vi "kuirs_LMS_滤除指定频率干扰_1.vi"() -> ()   [LabVIEW 2017]
uses:
  <vilib>/addons/Adaptive Filters/Create/AFT Create FIR LMS (Real).vi
  <vilib>/addons/Adaptive Filters/Processing/AFT Filter Signal and Update Coefficients (Real, Array).vi
  <vilib>/addons/Adaptive Filters/Analysis/AFT Get Coefficients (FIR, Real).vi
  <vilib>/Analysis/NI_AALBase.lvlib
  <vilib>/addons/Adaptive Filters/NI_AdaptiveFilter.lvlib
panel:
  out "max step":dbl
  out "coefficient":dbl[](graph)
  in  "干扰幅值":dbl(slide)=17.0 scale=0.1..2.0
  in  "噪声标准差":dbl(slide)=17.0 scale=0.0..3.0
  in  "信号周期":dbl(slide)=17.0 scale=0.0..10.0
  in  "停止按钮":bool
  in  "干扰周期":dbl(slide)=17.0 scale=0.0..40.0
  out "MIX SIGNAL":dbl[](graph)
  out "e(n)":dbl[](graph)
  out "LMS OUTPUT":dbl[](graph)
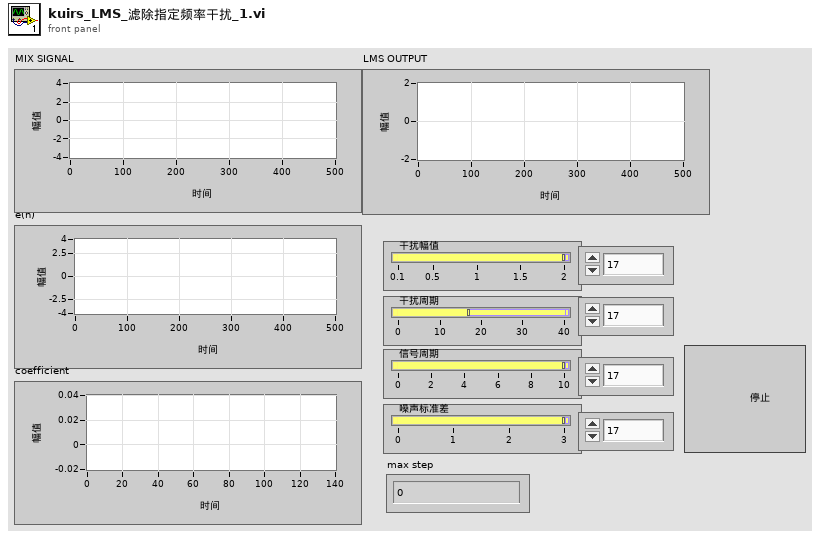
[diagram p1: front panel]
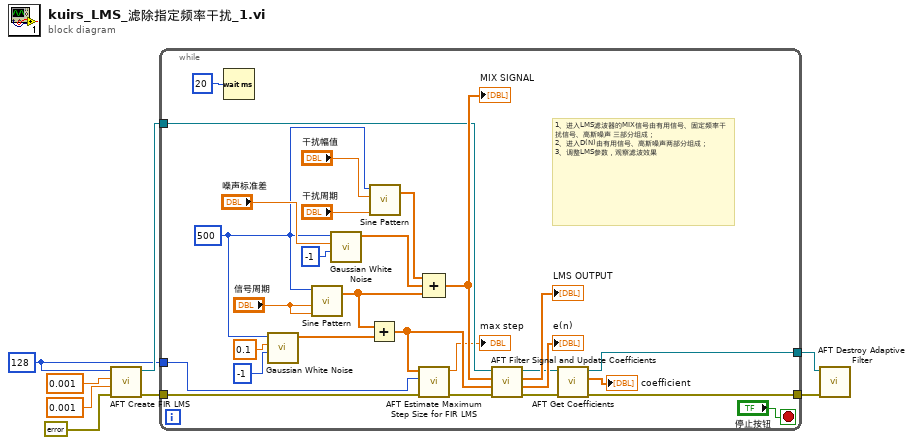
[diagram p0: block diagram]
diagram:
  w1 = 128 ("filter length")
  n1 = call-poly <vilib>:"AFT Create FIR LMS.vi"("error in (no error)"=errorcluster {"status"=FALSE, "code"=0, "source"=""}, "leakage"=0.001, "step size"=0.001, "filter length"=w1) -> ("error out"=w3:errorcluster, "adaptive filter out"=w6:refnum<k20>)  [unwired: 6 in]
  n2 = while {
    tunnel: w6 -> [w16]
    tunnel: [w23] -> w5
    tunnel: w3 -> [w18]
    tunnel: [w20] -> w4
    tunnel: w1 -> [w11]
    stop <- "停止按钮" stop-if-true
    w10 = 500 ("samples")
    # "1、进入LMS滤波器的MIX信号由有用信号、固定频率干扰信号、高斯噪声 三部分组成；\n2、进入D(N)由有用信号、高斯噪声两部分组成；\n3、调整LMS参数，观察滤波效果"
    n3 = Wait (ms)(milliseconds to wait=u32 20 ("等待时间（毫秒）")) -> ()  [unwired: 1 out]
    n4 = call <vilib>:"Gaussian White Noise.vi"("seed"=-1, "standard deviation"=0.1, "samples"=w10) -> ("Gaussian noise pattern"=w33:dbl[])  [unwired: 7 in, 1 out]
    n5 = call <vilib>:"Sine Pattern.vi"("cycles"="信号周期", "phase(degrees)"="信号周期", "samples"=w10) -> ("Sinusoidal Pattern"=w30:dbl[])  [unwired: 1 in, 1 out]
    n6 = call <vilib>:"Gaussian White Noise.vi"("seed"=-1, "standard deviation"="噪声标准差", "samples"=w10) -> ("Gaussian noise pattern"=w31:dbl[])  [unwired: 7 in, 1 out]
    n7 = Add(x=w30, y=w33) -> (x+y=w19:dbl[])
    n8 = call <vilib>:"Sine Pattern.vi"("cycles"="干扰周期", "amplitude"="干扰幅值", "samples"=w10) -> ("Sinusoidal Pattern"=w32:dbl[])  [unwired: 1 in, 1 out]
    n9 = call <vilib>:"AFT Estimate Maximum Step Size for FIR LMS.vi"("error in (no error)"=w18, "filter length"=w11, "x(n)"=w19) -> ("error out"=w17:errorcluster, "maximum step size"=→"max step":dbl)  [unwired: 7 in]
    n10 = Compound Arithmetic op=ADD(w32, w31, w30) -> (w34:dbl[])
    "MIX SIGNAL" <- w34
    n11 = call-poly <vilib>:"AFT Filter Signal and Update Coefficients.vi"("error in (no error)"=w17, "d(n)"=w19, "x(n)"=w34, "adaptive filter in"=w16) -> ("error out"=w21:errorcluster, "e(n)"=→"e(n)":dbl[], "y(n)"=→"LMS OUTPUT":dbl[], "adaptive filter out"=w24:refnum<k20>)  [unwired: 4 in]
    n12 = call-poly <vilib>:"AFT Get Coefficients.vi"("error in (no error)"=w21, "adaptive filter in"=w24) -> ("error out"=w20:errorcluster, "coefficients"=→"coefficient":dbl[], "adaptive filter out"=w23:refnum<k20>)  [unwired: 7 in]
  }
  n13 = call <vilib>:"AFT Destroy Adaptive Filter.vi"("error in (no error)"=w4, "adaptive filter in"=w5) -> ()  [unwired: 9 in, 1 out]
